vi "UpdateIO.vi"(11 "Count(ticks)":u32=20) -> ()   [LabVIEW 2012]
uses:
  <vilib>/eio/EIONode/EIONode.xnode
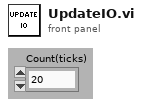
[diagram p1: front panel]
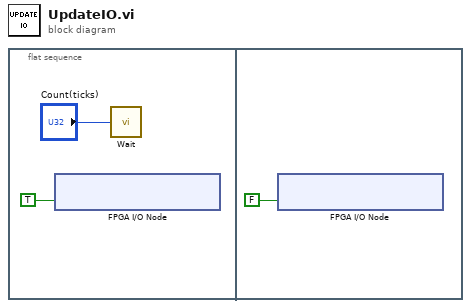
[diagram p0: block diagram]
diagram:
  n1 = flat-sequence {
    frame #0 {
      n2 = xnode "FPGA I/O Node"("IO Module\\UPDATE_IO"=TRUE ("IO Module\\UPDATE_IO")) -> ()  [unwired: 1 in, 1 out]
      n3 = call "Wait"("Count(Ticks)"="Count(ticks)") -> ()  [unwired: 1 out]
    }
    frame #1 {
      n4 = xnode "FPGA I/O Node"("IO Module\\UPDATE_IO"=FALSE ("IO Module\\UPDATE_IO")) -> ()  [unwired: 1 in, 1 out]
    }
  }
